vi "Put msg in mailbox2.vi"(8 "error in (no error)":errorcluster, 10 "Message":variant, 11 "Mailbox ref in":T1) -> (0 "error out":errorcluster, 2 "timed out?":bool, 3 "mailbox ref out":T1)   [LabVIEW 2021, in "MatS Libs.lvlib"]
uses:
  <userlib>/MatS Libs/MatS Libs.lvlib
  <userlib>/MatS Libs/MatS Mailman/TypeDefs/Mailbox ref.ctl
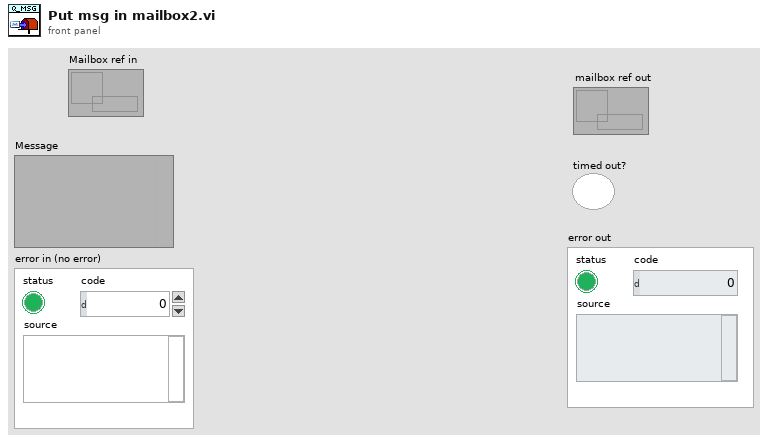
[diagram p1: front panel]
types:
  T1 = typedef "MatS Libs.lvlib/Mailbox ref.ctl" = refnum<queue>
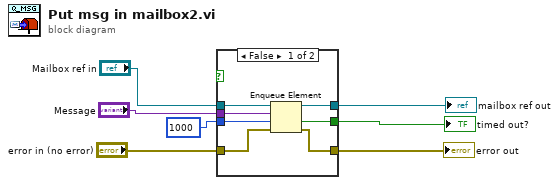
[diagram p0: block diagram]
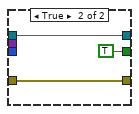
[diagram p2: hidden frame]
diagram:
  n1 = case shown="False" {
    selector: _ -> [_ _]
    tunnel: [w14 w17] -> w7
    tunnel: "Message" -> [w13 _]
    tunnel: "error in (no error)" -> [w12 w15]
    tunnel: 1000 ("timeout in ms (-1)") -> [w11 _]
    tunnel: [w10 TRUE ("timed out?")] -> w3
    tunnel: [w9 w15] -> w2
    tunnel: "Mailbox ref in" -> [w8 w17]
    frame False {
      n2 = Enqueue Element(queue=w8, element=w13, timeout in ms (-1)=w11, error in (no error)=w12) -> (queue out=w14:T1, timed out?=w10:bool, error out=w9:errorcluster)
    }
    frame True {
    }
  }
  "mailbox ref out" <- w7
  "timed out?" <- w3
  "error out" <- w2
